vi "DeadbandLimiter.vi"(0 "Deadband Percentage":dbl=0.1, 7 "Input":dbl) -> (8 "Deadband Output":dbl)   [LabVIEW 2018]
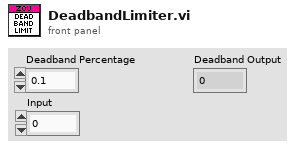
[diagram p1: front panel]
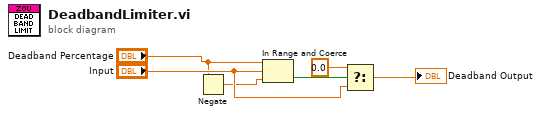
[diagram p0: block diagram]
diagram:
  n1 = Negate(x="Deadband Percentage") -> (-x=w2:dbl)
  n2 = In Range and Coerce(upper limit="Deadband Percentage", x="Input", lower limit=w2) -> (In Range?=w6:bool)  [unwired: 1 out]
  n3 = Select(t=0.0 ("f"), s=w6, f="Input") -> (s? t:f=→"Deadband Output":dbl)
